vi "GetCountAllTransactions.vi"() -> (1 "Pie Chart All data to user data":picture, 2 "Colors":u32[](array[colorbox])=[11796480, 37103, 40712, 16770816, 11796658, 4210752, 15517151], 3 "Pie Chart All Transactions":picture, 4 "Colors 2":u32[](array[colorbox])=[11796480, 37103, 40712, 16770816, 11796658, 4210752])   [LabVIEW 2014]
uses:
  USBAnalyzerEllisysDll.dll
panel:
  in  "return type":i32
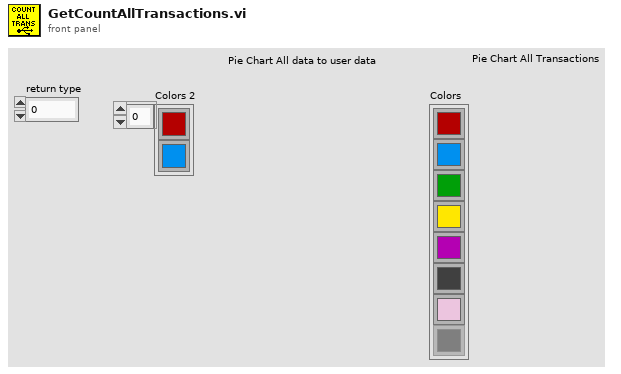
[diagram p1: front panel]
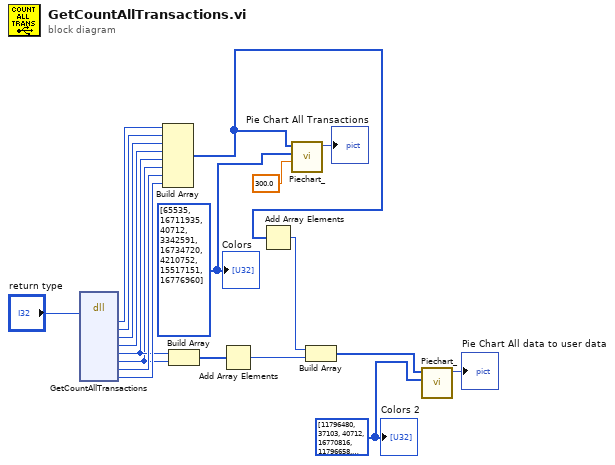
[diagram p0: block diagram]
diagram:
  w3 = u32[] [11796480, 37103, 40712, 16770816, 11796658, 4210752] ("Colors")
  w6 = u32[] [65535, 16711935, 40712, 3342591, 16734720, 4210752, 15517151, 16776960] ("Colors")
  n1 = dll-call lib="PTH2Wabs CUsersMichał\tDocumentsEllisysAnalyzerLabVIEWUSBAnalyzerEllisysDll.dll" fn="GetCountAllTransactions"("return type"="return type") -> ("in"=w8:u64, "out"=w9:u64, "setup"=w17:u64, "sof"=w18:u64, "data0"=w11:u64, "data1"=w10:u64, "ack"=w12:u64, "nak"=w16:u64)  [unwired: 11 in, 2 out]
  n2 = Build Array(w8, w9, w17, w18, w11, w10, w12, w16) -> (w7:u64[])
  n3 = Build Array(w11, w10) -> (w15:u64[])
  n4 = Add Array Elements(numeric array=w15) -> (sum=w13:u64)
  n5 = Add Array Elements(numeric array=w7) -> (sum=w14:u64)
  n6 = call "Piechart_.vi"("Pie Chart Size (200 pixels)"=300.0, "Division Colors"=w6, "Pie Chart Data (arb unit)"=w7) -> ("Pie Chart"=→"Pie Chart All Transactions":picture)  [unwired: 8 in]
  n7 = Build Array(w14, w13) -> (w4:u64[])
  n8 = call "Piechart_.vi"("Division Colors"=w3, "Pie Chart Data (arb unit)"=w4) -> ("Pie Chart"=→"Pie Chart All data to user data":picture)  [unwired: 9 in]
  "Colors" <- w6
  "Colors 2" <- w3
